vi "CRYUpdate Generator Index.vi"(8 "Chn Idx":i32, 10 "Gen_Index":i32) -> ()   [LabVIEW 2013]
uses:
  CRYMisc vis settings global.vi
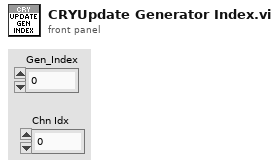
[diagram p1: front panel]
types:
  T1 = cluster{"Gen Idx":i32, "Chn Idx":i32, "Data":sgl[]}[]
  T2 = cluster{"Gen Idx":i32, "Chn Idx":i32, "Data":sgl[]}
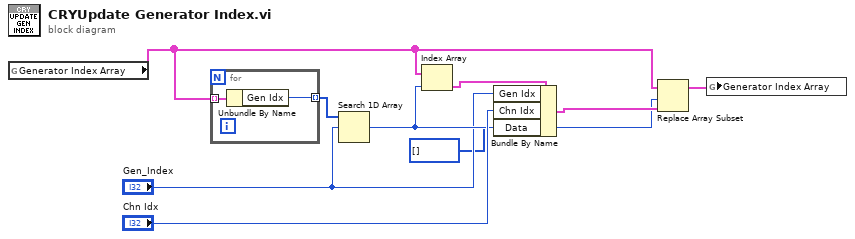
[diagram p0: block diagram]
diagram:
  n1 = global read "CRYMisc vis settings global.vi" "Generator Index Array"() -> (w4:T1)
  n2 = for {
    tunnel: w4 -> [w11] mode=indexing
    tunnel: [w10] -> w9 mode=indexing
    n3 = Unbundle By Name(w11) -> ("Gen Idx"=w10:i32)
  }
  n4 = Search 1D Array(1D array=w9, element="Gen_Index") -> (index of element=w5:i32)  [unwired: 1 in]
  n5 = Index Array(array=w4, index=w5) -> (element=w8:T2)
  n6 = Bundle By Name(cluster=w8, "Gen Idx"="Gen_Index", "Chn Idx"="Chn Idx", "Data"=i32[] []) -> (w6:T2)
  n7 = Replace Array Subset(array=w4, new element=w6, index=w5) -> (w3:T1)
  n8 = global write "CRYMisc vis settings global.vi" "Generator Index Array"(w3) -> ()
